vi "GEOM_ROIArr2Str.vi"(8 "error in (no error)":errorcluster) -> (0 "error out":errorcluster, 1 "ROI command":string, 2 "defined?":bool, 3 "nrois":i32, 4 "defined rois":string)   [LabVIEW 2016]
uses:
  GEOM_VAR_action.ctl
  GEOM_Gbls.vi
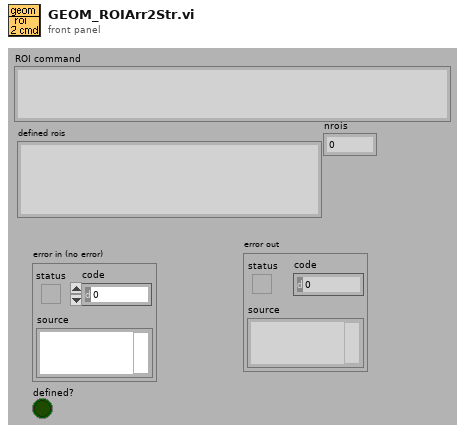
[diagram p1: front panel]
types:
  T1 = typedef "GEOM_VAR_action.ctl" = enum16{"read", "write"}
  T2 = typedef "GEOM_Coords.ctl" = cluster{"xstart":u32, "ystart":u32, "xsize":u32, "ysize":u32}
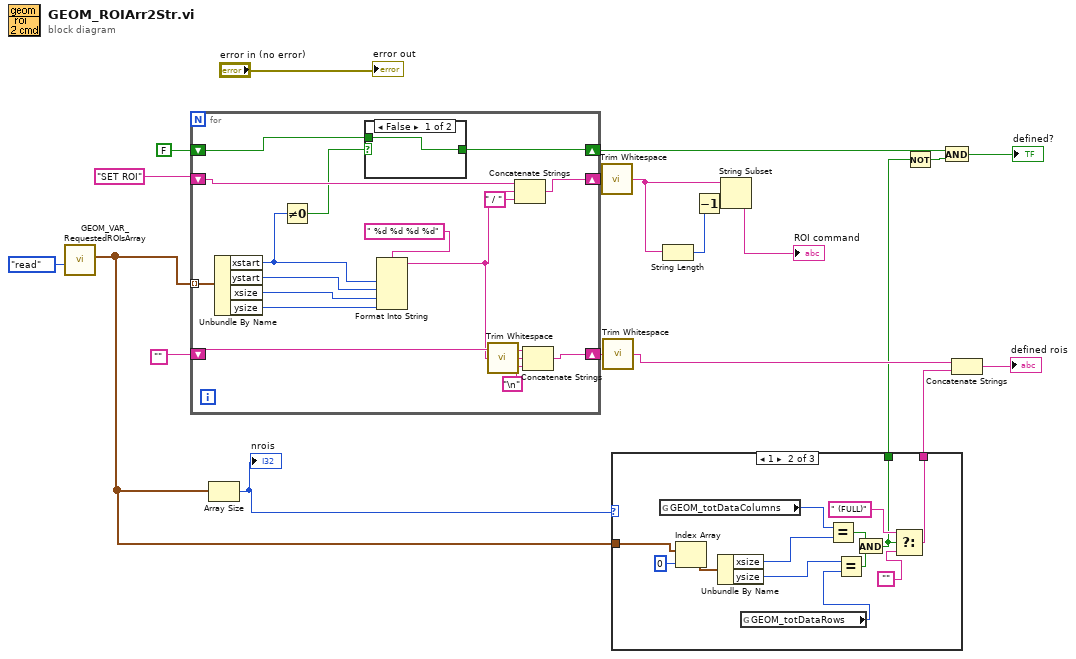
[diagram p0: block diagram]
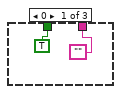
[diagram p2: hidden frame]
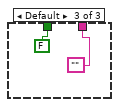
[diagram p3: hidden frame]
diagram:
  n1 = call "GEOM_VAR_RequestedROIsArray.vi"("Action"=GEOM_VAR_action."read") -> ("ROIs out"=w7:T2[])  [unwired: 1 in, 9 out]
  n2 = for {
    tunnel: w7 -> [w37] mode=indexing
    shift-right: [w32] -> w16
    shift-left: "SET ROI" ("format string") -> [w33]
    shift-right: [w29] -> w17
    shift-left: FALSE -> [w28]
    shift-right: [w23] -> w10
    shift-left: "" -> [w25]
    n3 = Unbundle By Name(w37) -> ("xstart"=w31:u32, "ystart"=w36:u32, "xsize"=w35:u32, "ysize"=w34:u32)
    n4 = Not Equal To 0?(x=w31) -> (x != 0?=w30:bool)
    n5 = case shown="False" w30 {
      selector: w30 -> [_ w39]
      tunnel: [w38 w39] -> w29
      tunnel: w28 -> [w38 _]
      frame False {
      }
      frame True {
      }
    }
    n6 = Format Into String(format string=" %d %d %d %d", w31, w36, w35, w34) -> (resulting string=w24:string)  [unwired: 2 in, 1 out]
    n7 = call <vilib>:"Trim Whitespace.vi"("string"=w24) -> ("trimmed string"=w21:string)  [unwired: 1 in]
    n8 = Concatenate Strings(w33, w24, " / " ("string")) -> (w32:string)
    n9 = Concatenate Strings(w25, w21, "\n") -> (w23:string)
  }
  n10 = Array Size(array=w7) -> (size(s)=w8:i32)
  "nrois" <- w8
  n11 = call <vilib>:"Trim Whitespace.vi"("string"=w16) -> ("trimmed string"=w9:string)  [unwired: 1 in]
  n12 = call <vilib>:"Trim Whitespace.vi"("string"=w10) -> ("trimmed string"=w6:string)  [unwired: 1 in]
  n13 = case shown="1" w8 {
    tunnel: w7 -> [_ w54 _]
    tunnel: ["" w43 ""] -> w5
    tunnel: [TRUE w42 FALSE] -> w2
    frame 0 {
    }
    frame 1 {
      n14 = global read "GEOM_Gbls.vi" "GEOM_totDataColumns"() -> (w48:u16)
      n15 = Index Array(array=w54, index=0) -> (element=w49:T2)
      n16 = Unbundle By Name(w49) -> ("xsize"=w47:u32, "ysize"=w46:u32)
      n17 = global read "GEOM_Gbls.vi" "GEOM_totDataRows"() -> (w45:u16)
      n18 = Equal?(x=w48, y=w47) -> (x = y?=w52:bool)
      n19 = Equal?(x=w46, y=w45) -> (x = y?=w51:bool)
      n20 = And(x=w52, y=w51) -> (x .and. y?=w42:bool)
      n21 = Select(t=" (FULL)", s=w42, f="") -> (s? t:f=w43:string)
    }
    frame Default {
    }
  }
  n22 = String Length(string=w9) -> (length=w15:i32)
  n23 = Decrement(x=w15) -> (x-1=w14:i32)
  n24 = String Subset(string=w9, length (rest)=w14) -> (substring=→"ROI command":string)  [unwired: 1 out]
  n25 = Not(x=w2) -> (.not. x?=w1:bool)
  n26 = And(x=w17, y=w1) -> (x .and. y?=→"defined?":bool)
  n27 = Concatenate Strings(w6, w5) -> (→"defined rois":string)
  "error out" <- "error in (no error)"
